vi "Load XML String.vi"(0 "XML string":string, 1 "preserve whitespace (True)":bool=TRUE, 2 "validate on load (Auto)":i32(ring)=2 items=["Never", "Always", "Auto"], 5 "process namespaces (False)":bool, 7 "process schema (False)":bool, 9 "load external DTD (True)":bool=TRUE, 11 "error in (no error)":errorcluster, 12 "schema full checking (False)":bool) -> (4 "DOM document out":refnum<k20>, 6 "parse errors":string, 15 "error out":errorcluster)   [LabVIEW 2017, in "NI_XML.lvlib"]
doc: "Opens an XML file and allows you to configure the XML parser to validate the file against a schema or Document Type Definition (DTD).\n\nNational Instruments recommends that you use the Close VI to close all the references after using the XML parser classes."
uses:
  <vilib>/xml/NI_XML.lvlib
  <resource>/objmgr/DOMUserDefRef.rc
panel:
  in  "error message":string="Empty XML string!"
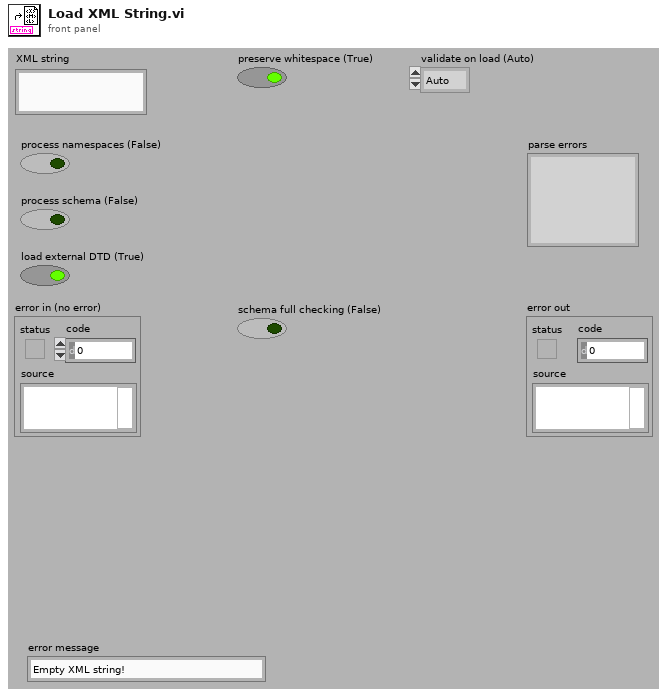
[diagram p1: front panel]
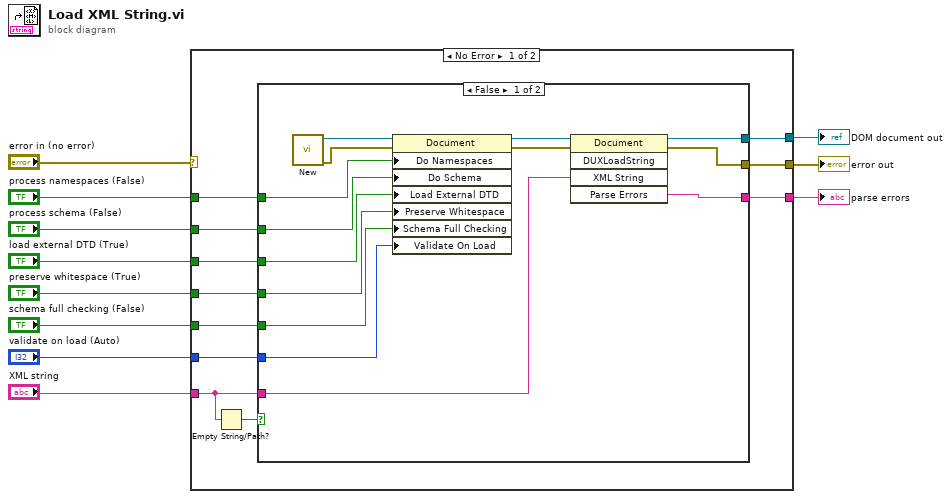
[diagram p0: block diagram]
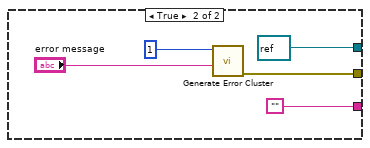
[diagram p2: hidden frame]
diagram:
  n1 = case shown="No Error" "error in (no error)" {
    selector: "error in (no error)" -> [_ w42]
    tunnel: [w21 _] -> w11
    tunnel: [w20 w42] -> w10
    tunnel: "XML string" -> [w19 _]
    tunnel: [w22 _] -> w7
    tunnel: "validate on load (Auto)" -> [w17 _]
    tunnel: "schema full checking (False)" -> [w16 _]
    tunnel: "preserve whitespace (True)" -> [w15 _]
    tunnel: "load external DTD (True)" -> [w14 _]
    tunnel: "process schema (False)" -> [w13 _]
    tunnel: "process namespaces (False)" -> [w12 _]
    frame No Error {
      n2 = Empty String/Path?(string/path=w19) -> (empty?=w18:bool)
      n3 = case shown="False" w18 {
        tunnel: [w36 ""] -> w22
        tunnel: [w31 refnum<k20> refnum ("DOM Document Out")] -> w21
        tunnel: [w30 w39] -> w20
        tunnel: w19 -> [w29 _]
        tunnel: w17 -> [w28 _]
        tunnel: w16 -> [w27 _]
        tunnel: w15 -> [w26 _]
        tunnel: w14 -> [w25 _]
        tunnel: w13 -> [w24 _]
        tunnel: w12 -> [w23 _]
        frame False {
          n4 = call <vilib>:"New.vi"() -> ("error out"=w34:errorcluster, "DOM document out"=w35:refnum<k20>)  [unwired: 1 in, 7 out]
          n5 = property class="Document"(reference=w35, error in=w34, "Do Namespaces"=w23, "Do Schema"=w24, "Load External DTD"=w25, "Preserve Whitespace"=w26, "Schema Full Checking"=w27, "Validate On Load"=w28) -> (reference out=w33:refnum<k20>, error out=w32:errorcluster)
          n6 = invoke class="Document" method="DUXLoadString"(reference=w33, error in=w32, "XML String"=w29) -> (reference out=w31:refnum<k20>, error out=w30:errorcluster, "Parse Errors"=w36:string)  [unwired: 2 in, 2 out]
        }
        frame True {
          n7 = call <vilib>:"Generate Error Cluster.vi"("Additional Message"="error message", "Code"=1) -> ("error out"=w39:errorcluster)  [unwired: 1 in, 8 out]
        }
      }
    }
    frame Error {
    }
  }
  "DOM document out" <- w11
  "error out" <- w10
  "parse errors" <- w7
